vi "SLL DI LV2 Global.vi"(6 "DI State Array":bool[](array[boolean]), 7 "Option":T2, 8 "error in (no error)":errorcluster, 9 "DI State":bool, 10 "DI Channel Name Array":T1[](array[typedef]), 11 "DI Channel Name":T1=enum."PS01TS") -> (0 "error out":errorcluster, 1 "Array of all DIs":T1[](array[typedef]), 2 "Digital Array Status":bool[](array[boolean]), 3 "Digital Line Status":bool)   [LabVIEW 2013]
uses:
  Controls/SLL DI Global Options.ctl
  Controls/SLL List of Digital Inputs.ctl
  Controls/ALTS-2015 LV2GBL Options.ctl
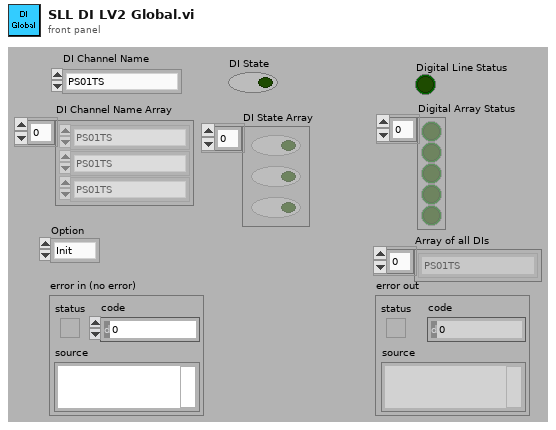
[diagram p1: front panel]
types:
  T1 = typedef "SLL List of Digital Inputs.ctl" = enum16{"MSSF", "MSSHC", "MSSMF", "MSSPRM", "MSSR", "PS01TS", "PX03TS", "PX04TS", "PX05TS", "PX06TS", "PX18TS", "READYTS"}
  T2 = typedef "SLL DI Global Options.ctl" = enum16{"Init", "Write Line", "Write Array", "Read Line", "Read Array", "Read Full Status", "Write Full Status"}
  T3 = typedef "ALTS-2015 LV2GBL Options.ctl" = enum16{"Read all", "Write all"}
  T4 = typedef "ALTS-2015 INI Configuration Cluster.ctl" = cluster{"Application":cluster{"Rerun Count":i32, "Workorder No":string}, "Station Details":cluster{"Sensor Name 1":string, "Sensor Name 2":string, "Sensor Name 3":string, "Sensor Name 4":string, "Station1 Enable":bool, "Station2 Enable":bool, "Station3 Enable":bool, "Station4 Enable":bool}, "Database":cluster{"Database Connection Link":path, "Result Procedure":string, "User":string, "Password":string, "Prompt":bool, "Station 1 LT Result DB DSN Path":path, "Station 2 LT Result DB DSN Path":path, "Station 3 LT Result DB DSN Path":path, "Station 4 LT Result DB DSN Path":path, "AirLeakTestResult Procedure":string, "Serial Details Procedure":string}, "Simulation":cluster{"Simulate DAQ Hardware":bool, "Simulate Result DB Write":bool, "Simulate Scanner":bool, "Simulate OPC":bool, "Simulate Serial Details DB":bool, "Simulate Result DB":bool, "Simulate Scanner DB Path":path, "Simulate Serial Details DB Path":path, "Simulate Result DB Path":path}, "Barcode Scanner1":cluster{"Scanner IP":string, "Scanner Port":u16, "#Bytes to Read":i32}, "Barcode Scanner2":cluster{"Enabled?":bool, "Scanner IP":string, "Scanner Port":u16, "#Bytes to Read":i32}}
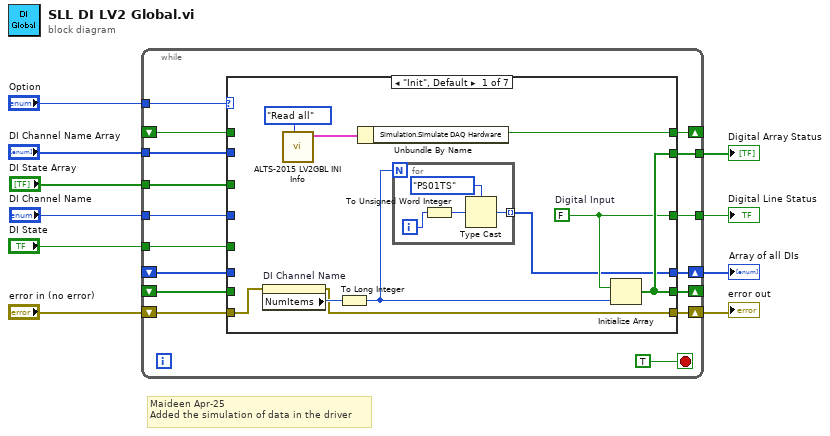
[diagram p0: block diagram]
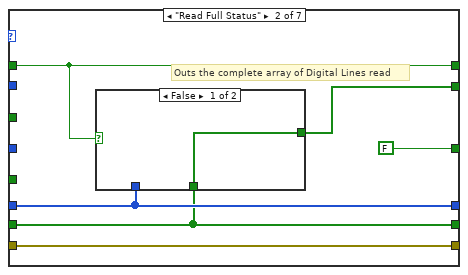
[diagram p2: hidden frame]
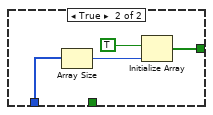
[diagram p3: hidden frame]
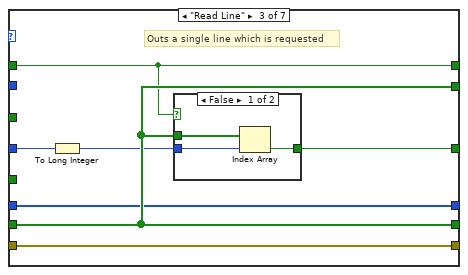
[diagram p4: hidden frame]
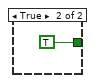
[diagram p5: hidden frame]
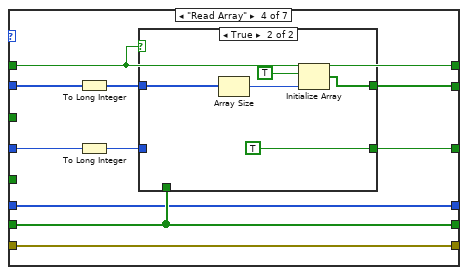
[diagram p6: hidden frame]
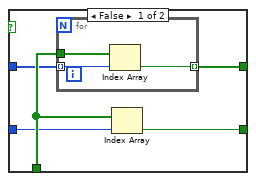
[diagram p7: hidden frame]
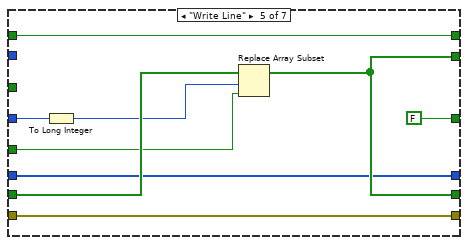
[diagram p8: hidden frame]
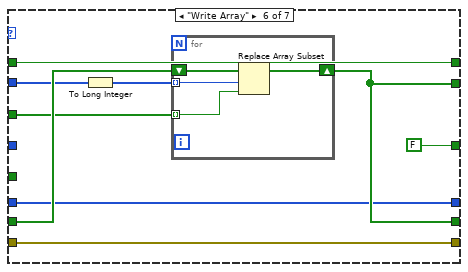
[diagram p9: hidden frame]
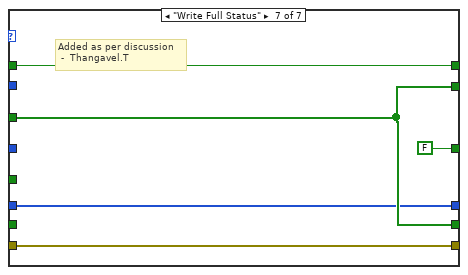
[diagram p10: hidden frame]
diagram:
  # "Maideen Apr-25\nAdded the simulation of data in the driver"
  n1 = while {
    shift-right: [w25] -> _
    shift-left: _ -> [w24]
    tunnel: "DI Channel Name Array" -> [w23]
    tunnel: "DI Channel Name" -> [w22]
    tunnel: [w21] -> w8
    tunnel: [w20] -> w7
    shift-right: [w18] -> w5
    shift-left: "error in (no error)" -> [w19]
    tunnel: "DI State Array" -> [w17]
    tunnel: "DI State" -> [w16]
    tunnel: "Option" -> [w15]
    shift-right: [w14] -> w1
    shift-left: _ -> [w13]
    shift-right: [w12] -> _
    shift-left: _ -> [w11]
    stop <- TRUE stop-if-true
    n2 = case shown="\"Init\", Default" w15 {
      tunnel: [w36 w41 w56 w69 w94 w103 w112] -> w25
      tunnel: w24 -> [_ w41 w56 w69 w91 w100 _]
      tunnel: w23 -> [_ _ _ w72 _ w98 _]
      tunnel: w22 -> [_ _ w58 w68 w89 _ _]
      tunnel: [w35 FALSE ("Digital Input") w57 w67 FALSE ("Digital Input") FALSE ("Digital Input") FALSE ("Digital Input")] -> w21
      tunnel: [w36 w42 w56 w71 w94 w103 w112] -> w20
      tunnel: w19 -> [w33 w45 w55 w70 w92 w101 w110]
      tunnel: [w32 w45 w55 w70 w92 w101 w110] -> w18
      tunnel: w17 -> [_ _ _ _ _ w99 w112]
      tunnel: w16 -> [_ _ _ _ w90 _ _]
      tunnel: [w30 w44 w53 w64 w87 w96 w111] -> w14
      tunnel: w13 -> [_ w44 w53 w64 w87 w96 w111]
      tunnel: [w27 w43 w52 w63 w86 w95 w108] -> w12
      tunnel: w11 -> [_ w43 w52 w63 w86 w95 w108]
      frame "Init", Default {
        w35 = FALSE  # Digital Input
        n3 = property on="DI Channel Name" class="Enum (strict)"(error in=w33) -> (error out=w32:errorcluster, "NumItems"=w34:u32)  [unwired: 1 in, 1 out]
        n4 = call "ALTS-2015 LV2GBL INI Info.vi"("Options"=ALTS-2015_LV2GBL_Options."Read all") -> ("Configuration Cluster Out"=w29:T4)  [unwired: 9 in, 1 out]
        n5 = To Long Integer(number=w34) -> (32bit integer=w31:i32)
        n6 = Unbundle By Name(w29) -> ("Simulation.Simulate DAQ Hardware"=w27:bool)
        n7 = for {
          N: w31 -> [_]
          tunnel: [w39] -> w30 mode=indexing
          i -> [w38]
          n8 = To Unsigned Word Integer(number=w38) -> (unsigned 16bit integer=w40:u16)
          n9 = Type Cast(type=SLL_List_of_Digital_Inputs."PS01TS" ("DI Channel Name"), x=w40) -> (*(type *) &x=w39:T1)
        }
        n10 = Initialize Array(w35, w31) -> (w36:bool[])
      }
      frame "Read Full Status" {
        # "Outs the complete array of Digital Lines read"
        n11 = case shown="False" w43 {
          tunnel: w44 -> [_ w51]
          tunnel: [w47 w48] -> w42
          tunnel: w41 -> [w47 _]
          frame False {
          }
          frame True {
            n12 = Array Size(array=w51) -> (size(s)=w50:i32)
            n13 = Initialize Array(TRUE ("Digital Input"), w50) -> (w48:bool[])
          }
        }
      }
      frame "Read Line" {
        # "Outs a single line which is requested"
        n14 = To Long Integer(number=w58) -> (32bit integer=w54:i32)
        n15 = case shown="False" w52 {
          tunnel: [w61 TRUE ("Digital Input")] -> w57
          tunnel: w56 -> [w60 _]
          tunnel: w54 -> [w59 _]
          frame False {
            n16 = Index Array(array=w60, index=w59) -> (element=w61:bool)
          }
          frame True {
          }
        }
      }
      frame "Read Array" {
        n17 = To Long Integer(number=w72) -> (32bit integer=w65:i32[])
        n18 = To Long Integer(number=w68) -> (32bit integer=w66:i32)
        n19 = case shown="True" w63 {
          tunnel: [w77 w81] -> w71
          tunnel: w69 -> [w76 _]
          tunnel: [w75 TRUE ("Digital Input")] -> w67
          tunnel: w66 -> [w74 _]
          tunnel: w65 -> [w73 w82]
          frame False {
            n20 = for {
              tunnel: w76 -> [w80]
              tunnel: w73 -> [w79] mode=indexing
              tunnel: [w78] -> w77 mode=indexing
              n21 = Index Array(array=w80, index=w79) -> (element=w78:bool)
            }
            n22 = Index Array(array=w76, index=w74) -> (element=w75:bool)
          }
          frame True {
            n23 = Array Size(array=w82) -> (size(s)=w84:i32)
            n24 = Initialize Array(TRUE ("Digital Input"), w84) -> (w81:bool[])
          }
        }
      }
      frame "Write Line" {
        n25 = To Long Integer(number=w89) -> (32bit integer=w88:i32)
        n26 = Replace Array Subset(array=w91, new element=w90, index=w88) -> (w94:bool[])
      }
      frame "Write Array" {
        n27 = To Long Integer(number=w98) -> (32bit integer=w97:i32[])
        n28 = for {
          tunnel: w99 -> [w105] mode=indexing
          shift-right: [w106] -> w103
          shift-left: w100 -> [w107]
          tunnel: w97 -> [w104] mode=indexing
          n29 = Replace Array Subset(array=w107, new element=w105, index=w104) -> (w106:bool[])
        }
      }
      frame "Write Full Status" {
        # "Added as per discussion\n -  Thangavel.T"
      }
    }
  }
  "error out" <- w5
  "Digital Line Status" <- w8
  "Digital Array Status" <- w7
  "Array of all DIs" <- w1
